vi "discrete_acquire_sequence.vi"(11 "Queue in":refnum<queue>) -> ()   [LabVIEW 2012]
uses:
  typedefs/MicroscopeEvent.ctl
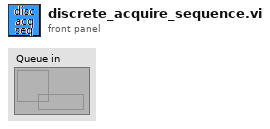
[diagram p1: front panel]
types:
  T1 = typedef "MicroscopeEvent.ctl" = enum16{"M.Wait", "M.RunRotation", "M.Flush", "M.Init", "M.InitStage", "M.InitImageData", "M.ReinitImageData", "M.ReinitImageParams", "M.GetSetParams", "M.InitFastHardware", "M.Pre-Acquire", "M.Acquire", "M.PostAcquire", "M.StopAcquire", "M.SetAcqStatusTrue", "M.SetAcqStatusFalse", "M.ClearImageData", "M.MoveStageDiscrete", "M.MoveStageToTarget1", "M.MoveStageToTarget2", "M.MoveStageToTarget3", "M.OpenShutters", "M.CloseShutters", "M.StartAcquireSequence", "M.ChangeParameters", "M.OpenStokes", "M.OpenPump", "M.RunSW"}
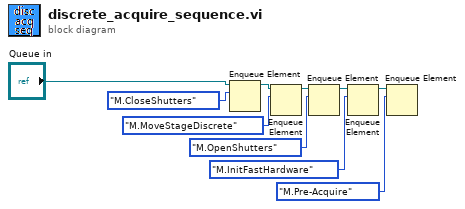
[diagram p0: block diagram]
diagram:
  n1 = Enqueue Element(queue="Queue in", element=MicroscopeEvent."M.CloseShutters") -> (queue out=w10:refnum<queue>)  [unwired: 2 in, 2 out]
  n2 = Enqueue Element(queue=w10, element=MicroscopeEvent."M.MoveStageDiscrete") -> (queue out=w7:refnum<queue>)  [unwired: 2 in, 2 out]
  n3 = Enqueue Element(queue=w7, element=MicroscopeEvent."M.OpenShutters") -> (queue out=w9:refnum<queue>)  [unwired: 2 in, 2 out]
  n4 = Enqueue Element(queue=w9, element=MicroscopeEvent."M.InitFastHardware") -> (queue out=w1:refnum<queue>)  [unwired: 2 in, 2 out]
  n5 = Enqueue Element(queue=w1, element=MicroscopeEvent."M.Pre-Acquire") -> ()  [unwired: 2 in, 3 out]
